vi "Handling DI param_ext.vi"(5 "initialise":bool, 6 "DP":bool[](array[boolean]), 7 "connect":bool[](array[boolean]), 8 "error in (no error)":errorcluster, 9 "DI":bool[][](array[boolean]), 10 "DIP":refnum<data-value>, 11 "DI short":T1) -> (0 "error out":errorcluster, 3 "DI out":T1)   [LabVIEW 2019, in "Inputs.lvlib"]
uses:
  Inputs.lvlib
  Ctl/DI short.ctl
  Ctl/Parameter State.ctl
  DI limits calc.vi
  Logik/fronts_ext.vi
  Trigers/RS32_ext.vi
  Timer Delay/DelayR_ext.vi
  Trigers/RS_ext.vi
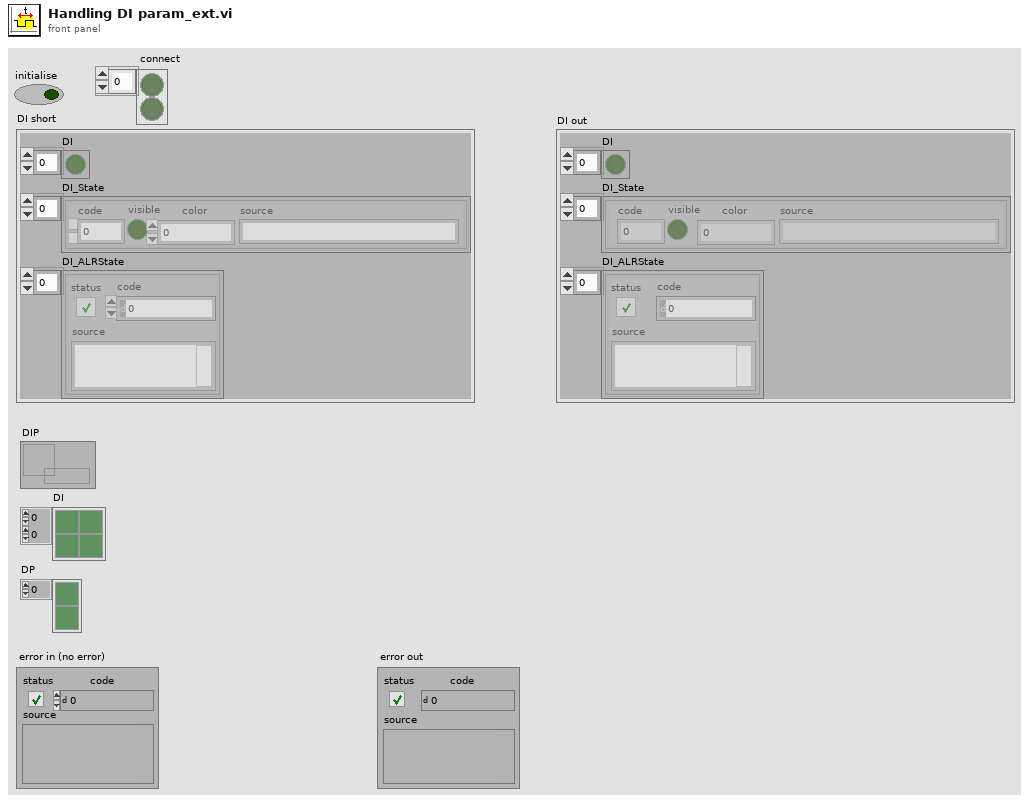
[diagram p1: front panel]
types:
  T1 = typedef "Inputs.lvlib/DI short.ctl" = cluster{"DI":bool[], "DI_State":T2[], "DI_ALRState":errorcluster[]}
  T2 = typedef "Inputs.lvlib/Parameter State.ctl" = cluster{"code":i32, "visible":bool, "color":u32, "source":string}
  T3 = cluster{"fronts not in":bool, "DelayR reg":cluster{"not in":bool, "T old":u32, "out":bool, "Q":bool}, "RS32 Q":u32}[]
  T4 = cluster{"fronts not in":bool, "DelayR reg":cluster{"not in":bool, "T old":u32, "out":bool, "Q":bool}, "RS32 Q":u32}
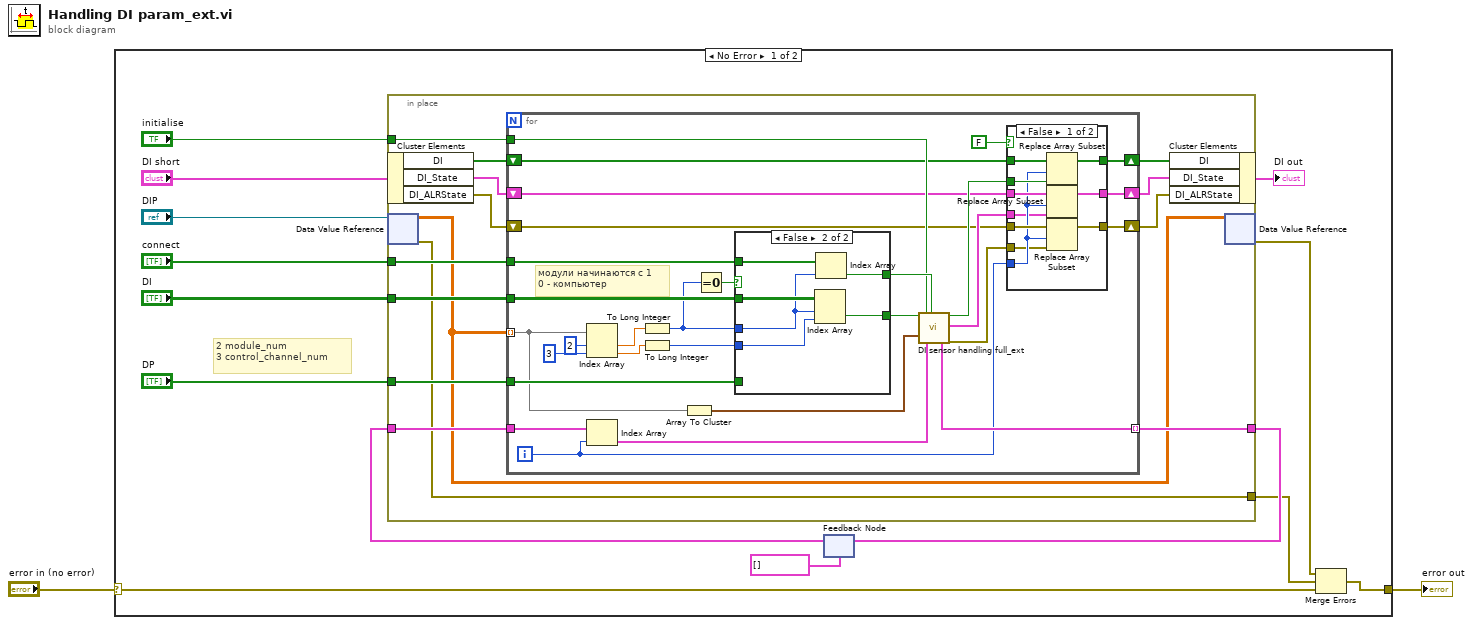
[diagram p0: block diagram]
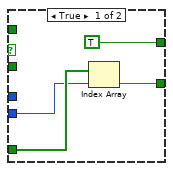
[diagram p2: hidden frame]
diagram:
  n1 = case shown="No Error" "error in (no error)" {
    selector: "error in (no error)" -> [w5 w83]
    tunnel: [w4 w83] -> w1
    frame No Error {
      # "2 module_num\n3 control_channel_num"
      n2 = feedback #1(T3 []) -> (w11:T3)
      n3 = in-place {
        in-place-border: "initialise" -> [w30]
        in-place-border: "connect" -> [w29]
        in-place-border: "DI" -> [w28]
        in-place-border: "DP" -> [w27]
        in-place-border: [w26] -> w12
        in-place-border: w11 -> [w25]
        in-place-border: [w18] -> w6
        n4 = in-place-cluster #2("DI short") -> ("DI"=w24:bool[], "DI_State"=w23:T2[], "DI_ALRState"=w22:errorcluster[])
        n5 = in-place-dvr #3("DIP") -> (w17:dbl[][], w18:errorcluster)
        n6 = for {
          tunnel: w17 -> [w44] mode=indexing
          tunnel: w28 -> [w52]
          tunnel: w29 -> [w54]
          tunnel: w30 -> [w41]
          tunnel: w27 -> [w49]
          tunnel: [w40] -> w26 mode=indexing
          tunnel: w25 -> [w38]
          shift-right: [w35] -> w21
          shift-left: w24 -> [w39]
          shift-right: [w34] -> w20
          shift-left: w23 -> [w33]
          shift-right: [w31] -> w19
          shift-left: w22 -> [w32]
          i -> [w37]
          # "модули начинаются с 1\n0 - компьютер"
          n7 = Index Array(array=w44, index #1=2 ("index (col)"), index #2=3 ("index (col)")) -> (element #1=w56:dbl, element #2=w55:dbl)
          n8 = Index Array(array=w38, index=w37) -> (element=w36:T4)
          n9 = To Long Integer(number=w56) -> (32bit integer=w51:i32)
          n10 = To Long Integer(number=w55) -> (32bit integer=w50:i32)
          n11 = Array To Cluster(array=w44) -> (cluster=w43:cluster{"[0]":dbl, "[1]":dbl})
          n12 = Equal To 0?(x=w51) -> (x = 0?=w53:bool)
          n13 = case shown="False" w53 {
            tunnel: w52 -> [_ w69]
            tunnel: w54 -> [_ w68]
            tunnel: w51 -> [_ w66]
            tunnel: w50 -> [w62 w67]
            tunnel: w49 -> [w63 _]
            tunnel: [TRUE ("Boolean") w65] -> w48
            tunnel: [w60 w64] -> w42
            frame True {
              n14 = Index Array(array=w63, index=w62) -> (element=w60:bool)
            }
            frame False {
              n15 = Index Array(array=w69, index (row)=w66, index (col)=w67) -> (element=w64:bool)
              n16 = Index Array(array=w68, index=w66) -> (element=w65:bool)
            }
          }
          n17 = call "DI sensor handling full_ext.vi"("DI"=w42, "control"=w43, "initialise"=w41, "DI sensor handling full reg old"=w36, "connect"=w48) -> ("DI sensor handling full reg"=w40:T4, "DIOUT"=w47:bool, "STATE"=w46:T2, "ALRSTATE"=w45:errorcluster)  [unwired: 9 in, 2 out]
          n18 = case shown="False" FALSE {
            tunnel: w46 -> [w71 _]
            tunnel: w47 -> [w79 _]
            tunnel: w37 -> [w72 _]
            tunnel: w45 -> [w70 _]
            tunnel: w39 -> [w78 w82]
            tunnel: [w77 w82] -> w35
            tunnel: [w76 w80] -> w34
            tunnel: w33 -> [w75 w80]
            tunnel: w32 -> [w74 w81]
            tunnel: [w73 w81] -> w31
            frame False {
              n19 = Replace Array Subset(array=w78, new element=w79, index=w72) -> (w77:bool[])
              n20 = Replace Array Subset(array=w75, new element=w71, index=w72) -> (w76:T2[])
              n21 = Replace Array Subset(array=w74, new element=w70, index=w72) -> (w73:errorcluster[])
            }
            frame True {
            }
          }
        }
        n22 = in-place-cluster #2("DI"=w21, "DI_State"=w20, "DI_ALRState"=w19) -> (→"DI out":T1)
        n23 = in-place-dvr #3(w17) -> (w7:errorcluster)  [unwired: 1 out]
      }
      n24 = feedback-in #1(w12) -> ()
      n25 = Merge Errors(w7, w6, w5) -> (w4:errorcluster)
    }
    frame Error {
    }
  }
  "error out" <- w1
